vi "TLPM Get Power Autorange Mode.vi"(8 "error in (no error)":errorcluster {"code" format="%.0x"}, 11 "instrument handle":refnum<visa-resource-name>) -> (0 "error out":errorcluster {"code" format="%.0x"}, 2 "Power Autorange Mode":bool, 3 "instrument handle out":refnum<visa-resource-name>)   [LabVIEW 2019]
doc: "This VI returns the power auto range mode."
uses:
  TLPM_32.dll
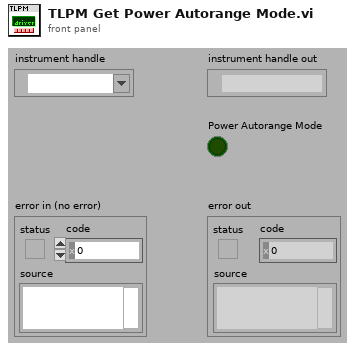
[diagram p1: front panel]
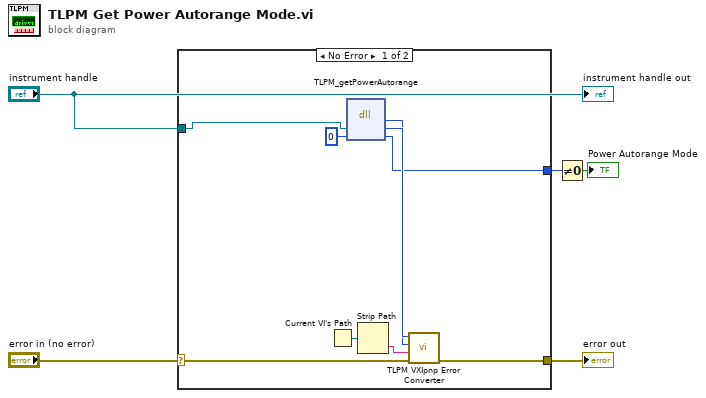
[diagram p0: block diagram]
diagram:
  n1 = case shown="No Error" "error in (no error)" {
    selector: "error in (no error)" -> [w9 w15]
    tunnel: [w8 w15] -> w5
    tunnel: "instrument handle" -> [w13 _]
    tunnel: [w6 _] -> w1
    frame No Error {
      n2 = Current VI's Path() -> (path=w14:path)
      n3 = dll-call lib="TLPM_32.dll" fn="TLPM_getPowerAutorange"("Instrument Handle"=w13, "Power Autorange Mode"=i16 0) -> (w11:i32, "Instrument Handle"=w12:u32, "Power Autorange Mode"=w6:i16)  [unwired: 3 in, 2 out]
      n4 = Strip Path(path=w14) -> (name=w10:string)  [unwired: 1 out]
      n5 = call <userlib>:"TLPM VXIpnp Error Converter.vi"("error in (no error)"=w9, "Name Of VI (\"\")"=w10, "CVI Error Code (0)"=w11, "instrument handle"=w12) -> ("error out"=w8:errorcluster)  [unwired: 6 in, 1 out]
    }
    frame Error {
    }
  }
  "error out" <- w5
  n6 = Not Equal To 0?(x=w1) -> (x != 0?=→"Power Autorange Mode":bool)
  "instrument handle out" <- "instrument handle"
